vi "Untitled 1.vi"() -> ()   [LabVIEW 2025]
uses:
  <vilib>/Utility/error.llb/DialogType.ctl
  channel parameters cluster.ctl
  <resource>/objmgr/daqmx.rc
  <vilib>/DAQmx/write.llb/DAQmx Write (Analog 1D Wfm NChan NSamp).vi
  <vilib>/DAQmx/write.llb/DAQmx Write (Analog 1D DBL NChan 1Samp).vi
panel:
  in  "Galvo voltage":dbl
  in  "Galvo frequency":u16
  in  "Pulse Duty Cycle":dbl
  in  "Zelux Frequency":u16
  in  "488 nm LED control":dbl(slide) step=1.0 scale=0.0..100.0 scale format="%#_3g"
  in  "594 nm laser control":dbl(slide) step=1.0 scale=0.0..100.0 scale format="%#_3g"
  in  "Run Live":bool caption="Run live"
  out "594 changed":bool=TRUE
  out "488 changed":bool=TRUE
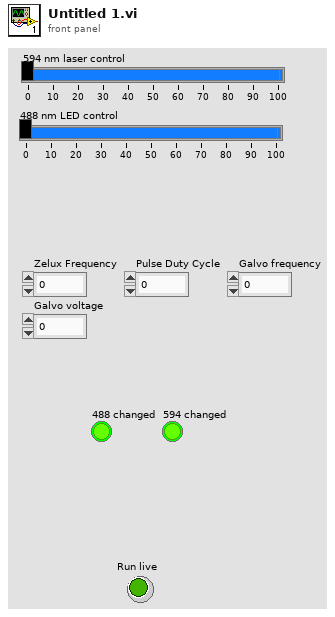
[diagram p1: front panel]
types:
  T1 = typedef "DialogType.ctl" = u16
  T2 = typedef "channel parameters cluster.ctl" = cluster{"voltage":dbl, "frequency":dbl, "duty cycle":dbl, "sample rate":dbl}
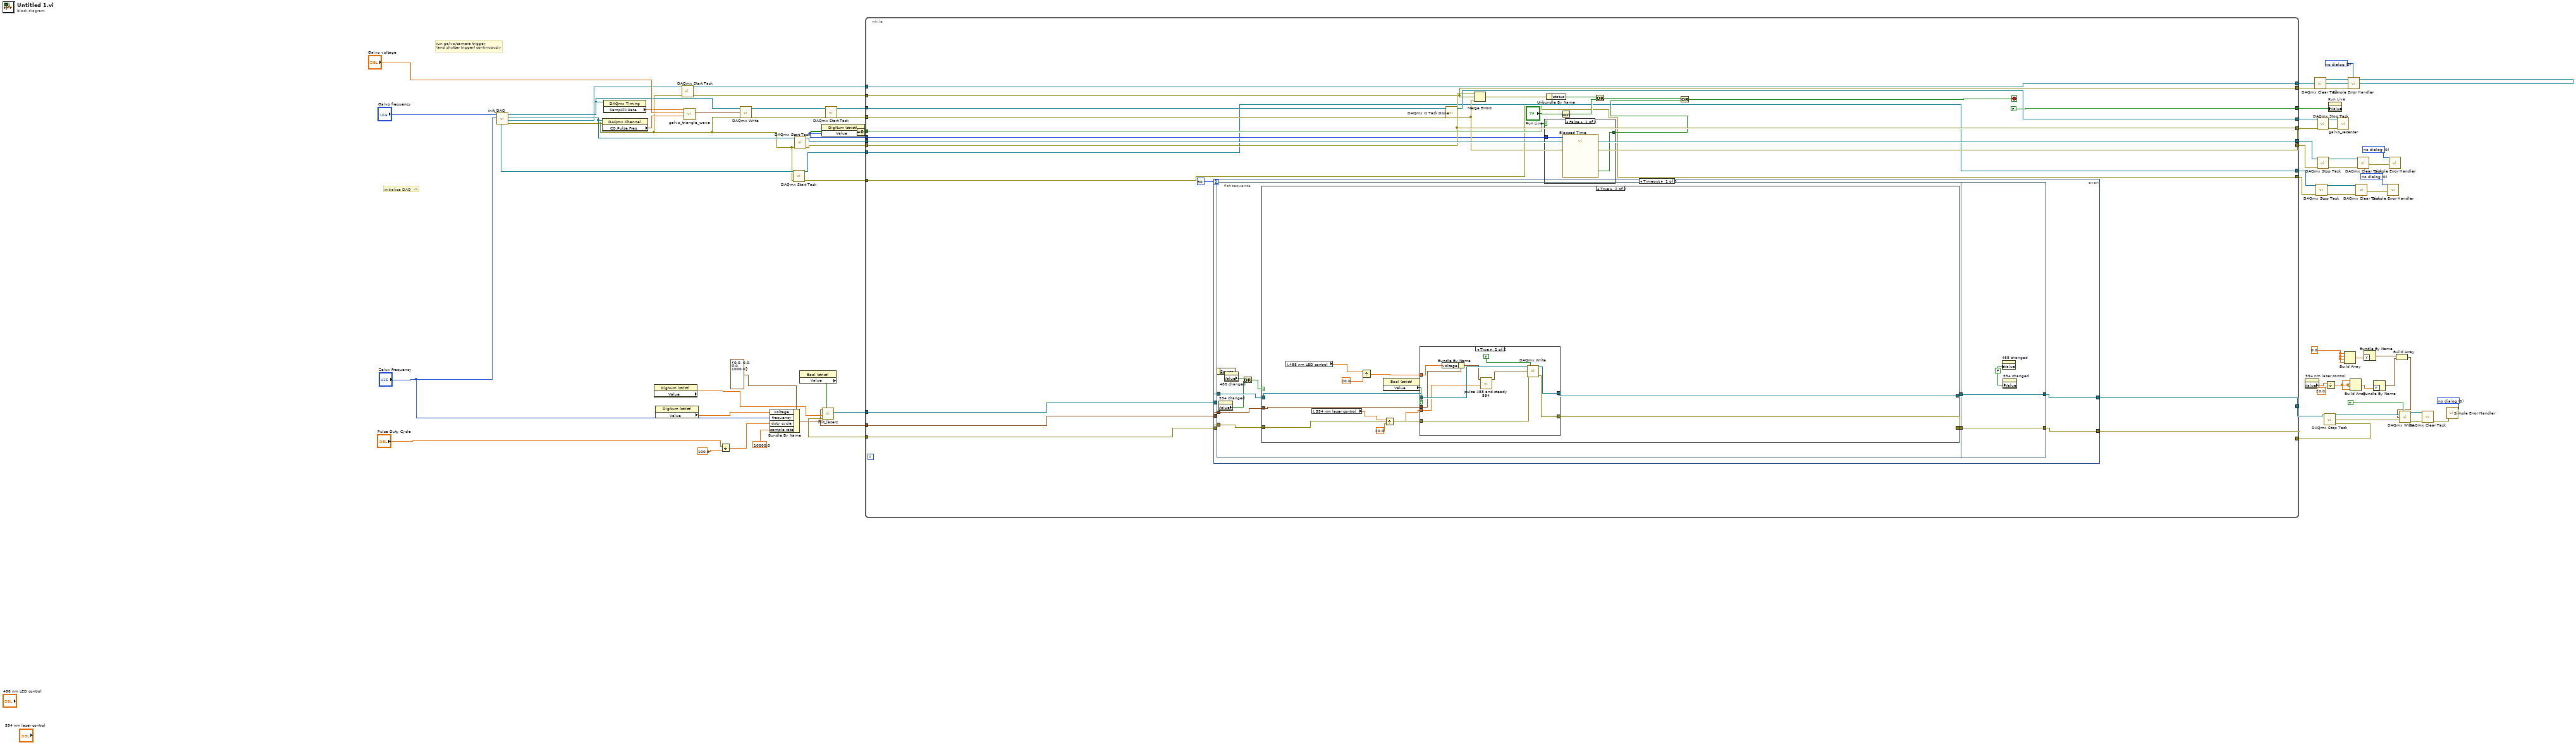
[diagram p0: block diagram]
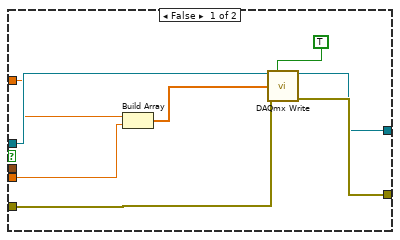
[diagram p3: hidden frame]
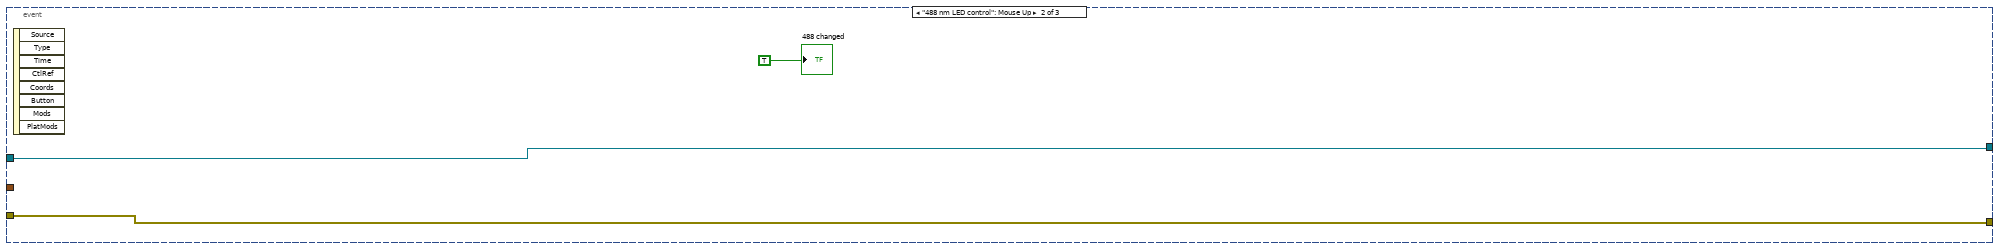
[diagram p4: hidden frame]
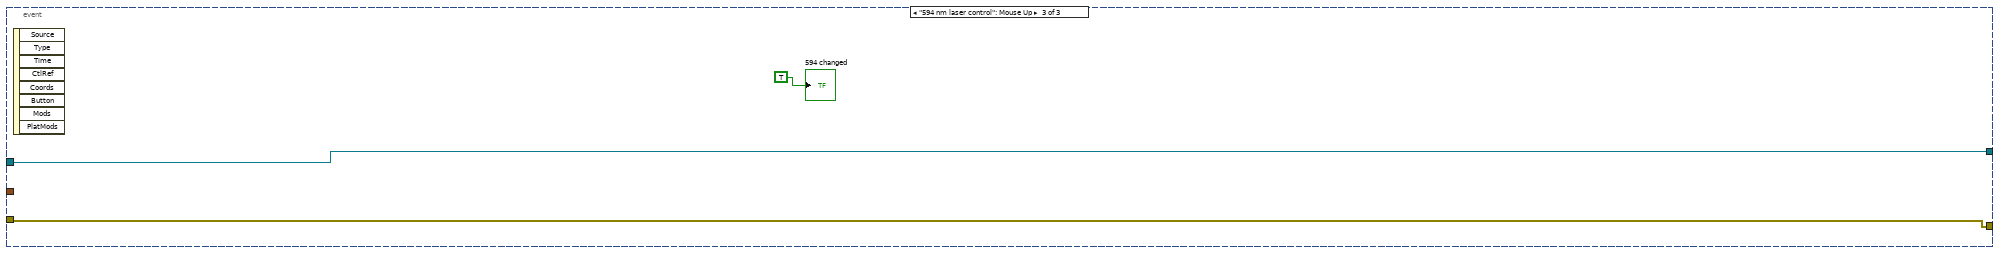
[diagram p5: hidden frame]
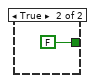
[diagram p6: hidden frame]
diagram:
  w5 = T1 0 items=["no dialog", "OK message", "continue or stop message", "OK message + warnings", "continue/stop + warnings"] ("type of dialog (OK msg:1)")
  w16 = 0.0
  w32 = T1 0 items=["no dialog", "OK message", "continue or stop message", "OK message + warnings", "continue/stop + warnings"] ("type of dialog (OK msg:1)")
  w57 = T1 0 items=["no dialog", "OK message", "continue or stop message", "OK message + warnings", "continue/stop + warnings"] ("type of dialog (OK msg:1)")
  w59 = T1 0 items=["no dialog", "OK message", "continue or stop message", "OK message + warnings", "continue/stop + warnings"] ("type of dialog (OK msg:1)")
  # "initialize DAQ  ->"
  # "run galvo/camera trigger \n(and shutter trigger) continuously"
  n1 = call "init_DAQ.vi"("Slow/Zelux frame frequency"="Zelux Frequency", "Fast/Kinetix frame frequency"="Galvo frequency") -> ("error out"=w9:errorcluster, "shutter trigger task"=w52:refnum<k21>, "Kinetix trigger task"=w47:refnum<k21>, "galvo driving task"=w63:refnum<k21>, "Zelux trigger task"=w10:refnum<k21>)  [unwired: 3 in, 2 out]
  n2 = property class="DAQmx Channel"(reference=w47, error in=w9) -> ("CO.Pulse.Freq"=w40:dbl)  [unwired: 2 out]
  n3 = property class="DAQmx Timing"(reference=w63) -> ("SampClk.Rate"=w39:dbl)  [unwired: 1 in, 2 out]
  n4 = property on="Property Node" class="DigNum (strict)"() -> ("Value"=w21:dbl)  [unwired: 2 in, 2 out]
  n5 = property on="Property Node" class="DigNum (strict)"() -> ("Value"=w22:dbl)  [unwired: 2 in, 2 out]
  n6 = call <vilib>:"DAQmx Start Task.vi"("task/channels in"=w52, "error in"=w9) -> ("task out"=w56:refnum<k21>, "error out"=w54:errorcluster)  [unwired: 12 in]
  n7 = call "galvo_triangle_wave.vi"("final frequency"=w40, "amplitude"="Galvo voltage", "sample rate"=w39) -> ("waveform array out"=w46:waveform(dbl)[])  [unwired: 8 in]
  n8 = Divide(x="Pulse Duty Cycle", y=100.0) -> (x/y=w25:dbl)
  n9 = call-poly <vilib>:"DAQmx Write.vi"("task/channels in"=w63, "data"=w46, "error in"=w9) -> ("task out"=w69:refnum<k21>, "error out"=w68:errorcluster)  [unwired: 10 in, 1 out]
  n10 = Bundle By Name(cluster=T2 {"voltage"=0.0, "frequency"=0.0, "duty cycle"=0.0, "sample rate"=1000.0} ("channel parameters"), "voltage"=w22, "frequency"="Zelux Frequency", "duty cycle"=w25, "sample rate"=10000.0) -> (w20:T2)
  n11 = call <vilib>:"DAQmx Start Task.vi"("task/channels in"=w10, "error in"=w9) -> ("task out"=w8:refnum<k21>, "error out"=w7:errorcluster)  [unwired: 12 in]
  n12 = call <vilib>:"DAQmx Start Task.vi"("task/channels in"=w47, "error in"=w9) -> ("task out"=w62:refnum<k21>, "error out"=w61:errorcluster)  [unwired: 12 in]
  n13 = property on="Property Node" class="Bool (strict)"() -> ("Value"=w27:bool)  [unwired: 2 in, 2 out]
  n14 = property on="Property Node" class="DigNum (strict)"() -> ("Value"=w42:i32)  [unwired: 2 in, 2 out]
  n15 = call "init_lasers.vi"("488 pulsed"=w27, "594 nm voltage"=w21, "488 nm channel parameters"=w20) -> ("error out"=w37:errorcluster, "task out"=w38:refnum<k21>)  [unwired: 6 in, 1 out]
  n16 = call <vilib>:"DAQmx Start Task.vi"("task/channels in"=w69, "error in"=w68) -> ("task out"=w64:refnum<k21>, "error out"=w65:errorcluster)  [unwired: 12 in]
  n17 = Equal To 0?(x=w42) -> (x = 0?=w43:bool)
  n18 = while {
    tunnel: w64 -> [w99]
    tunnel: w65 -> [w98]
    tunnel: [w88] -> w67
    tunnel: [w97] -> w66
    tunnel: w62 -> [w95]
    tunnel: w61 -> [w90]
    tunnel: [w90] -> w51
    tunnel: [w95] -> w49
    tunnel: w56 -> [w92]
    tunnel: [w92] -> w55
    tunnel: w54 -> [w89]
    tunnel: [w89] -> w53
    tunnel: w43 -> [w84]
    tunnel: w42 -> [w83]
    tunnel: [FALSE] -> w41
    tunnel: w38 -> [w81]
    tunnel: w37 -> [w80]
    tunnel: [w79] -> w36
    tunnel: [w78] -> w35
    tunnel: w20 -> [w76]
    tunnel: [w75] -> w2
    tunnel: w8 -> [w75]
    tunnel: [w74] -> w1
    tunnel: w7 -> [w74]
    stop <- w82 stop-if-true
    n19 = event shown="[0] Timeout" {
      selector: _ -> [_ _ _]
      dyn-events: _ -> [_ _ _]
      timeout: 50 -> [_ _ _]
      tunnel: w80 -> [w106 w151 w154]
      tunnel: [w100 w150 w153] -> w79
      tunnel: [w105 w151 w154] -> w78
      tunnel: w81 -> [w104 w150 w153]
      tunnel: w76 -> [w103 _ _]
      event Timeout {
        n20 = flat-sequence {
          tunnel: w106 -> [w114]
          tunnel: w104 -> [w112]
          tunnel: w103 -> [w107]
          tunnel: [w113] -> w102
          tunnel: [w108] -> w101
          tunnel: [w148] -> w100
          tunnel: [w149] -> w105
          tunnel: w102 -> [w149]
          tunnel: w101 -> [w148]
          frame #0 {
            n21 = property on="594 changed" class="Bool (strict)"() -> ("Value"=w109:bool)  [unwired: 2 in, 2 out]
            n22 = property on="488 changed" class="Bool (strict)"() -> ("Value"=w110:bool)  [unwired: 2 in, 2 out]
            n23 = Or(x=w110, y=w109) -> (x .or. y?=w111:bool)
            n24 = case shown="True" w111 {
              tunnel: w114 -> [w116 w127]
              tunnel: [w115 w126] -> w108
              tunnel: [w116 w125] -> w113
              tunnel: w112 -> [w115 w122]
              tunnel: w107 -> [_ w119]
              frame False {
              }
              frame True {
                n25 = local read "488 nm LED control"() -> (w118:dbl)
                n26 = local read "594 nm laser control"() -> (w117:dbl)
                n27 = Divide(x=w118, y=20.0) -> (x/y=w124:dbl)
                n28 = property on="Property Node" class="Bool (strict)"() -> ("Value"=w128:bool)  [unwired: 2 in, 2 out]
                n29 = Divide(x=w117, y=20.0) -> (x/y=w123:dbl)
                n30 = case shown="True" w128 {
                  tunnel: [w136 w143] -> w125
                  tunnel: w127 -> [w135 w144]
                  tunnel: w122 -> [w133 w145]
                  tunnel: [w134 w146] -> w126
                  tunnel: w124 -> [w131 w139]
                  tunnel: w123 -> [w130 w141]
                  tunnel: w119 -> [_ w138]
                  frame False {
                    n31 = Build Array(w131, w130) -> (w129:dbl[])
                    n32 = call-poly <vilib>:"DAQmx Write.vi"("task/channels in"=w133, "auto start"=TRUE, "data"=w129, "error in"=w135) -> ("task out"=w134:refnum<k21>, "error out"=w136:errorcluster)  [unwired: 9 in, 1 out]
                  }
                  frame True {
                    n33 = Bundle By Name(cluster=w138, "voltage"=w139) -> (w137:T2)
                    n34 = call "pulse 488 and steady 594.vi"("594 amplitude"=w141, "488 nm channel parameters"=w137) -> ("waveforms out"=w140:waveform(dbl)[])  [unwired: 9 in]
                    n35 = call-poly <vilib>:"DAQmx Write.vi"("task/channels in"=w145, "auto start"=TRUE, "data"=w140, "error in"=w144) -> ("task out"=w146:refnum<k21>, "error out"=w143:errorcluster)  [unwired: 9 in, 1 out]
                  }
                }
              }
            }
          }
          frame #1 {
            w147 = FALSE ("488 changed")
            n36 = property on="488 changed" class="Bool (strict)"("Value"=w147) -> ()  [unwired: 2 in, 2 out]
            n37 = property on="594 changed" class="Bool (strict)"("Value"=w147) -> ()  [unwired: 2 in, 2 out]
          }
        }
        n38 = event-data() -> ()  [unwired: 1 in, 1 out]
      }
      event "488 nm LED control": Mouse Up {
        n39 = event-data() -> ()  [unwired: 1 in, 8 out]
        "488 changed" <- TRUE ("488 changed")
      }
      event "594 nm laser control": Mouse Up {
        n40 = event-data() -> ()  [unwired: 1 in, 8 out]
        "594 changed" <- TRUE
      }
    }
    n41 = call <vilib>:"DAQmx Is Task Done.vi"("task/channels in"=w99, "error in"=w98) -> ("task out"=w97:refnum<k21>, "error out"=w88:errorcluster)  [unwired: 11 in, 1 out]
    n42 = Merge Errors(w90, w89, w88) -> (w91:errorcluster)
    n43 = case shown="False" w84 {
      tunnel: [w157 FALSE] -> w86
      tunnel: w83 -> [w156 _]
      frame False {
        n44 = call "Elapsed Time"("Time Target (s)"=w156) -> ("Time has Elapsed"=w157:bool)  [unwired: 11 in, 7 out]
      }
      frame True {
      }
    }
    n45 = Unbundle By Name(w91) -> ("status"=w96:bool)
    n46 = Not(x="Run Live") -> (.not. x?=w94:bool)
    n47 = Or(x=w96, y=w94) -> (x .or. y?=w87:bool)
    n48 = Or(x=w87, y=w86) -> (x .or. y?=w82:bool)
  }
  n49 = property on="594 nm laser control" class="Slide (strict)"() -> ("Value"=w15:dbl)  [unwired: 2 in, 2 out]
  n50 = call <vilib>:"DAQmx Clear Task.vi"("task in"=w55, "error in"=w53) -> ("error out"=w58:errorcluster)  [unwired: 13 in]
  n51 = call <vilib>:"DAQmx Stop Task.vi"("task/channels in"=w2, "error in"=w1) -> ("task out"=w3:refnum<k21>, "error out"=w4:errorcluster)  [unwired: 12 in]
  n52 = call <vilib>:"DAQmx Stop Task.vi"("task/channels in"=w66, "error in"=w67) -> ("task out"=w45:refnum<k21>, "error out"=w44:errorcluster)  [unwired: 12 in]
  n53 = call <vilib>:"DAQmx Stop Task.vi"("task/channels in"=w49, "error in"=w51) -> ("task out"=w48:refnum<k21>, "error out"=w50:errorcluster)  [unwired: 12 in]
  n54 = call <vilib>:"DAQmx Stop Task.vi"("task/channels in"=w36, "error in"=w35) -> ("task out"=w33:refnum<k21>, "error out"=w34:errorcluster)  [unwired: 12 in]
  n55 = Divide(x=w15, y=20.0) -> (x/y=w13:dbl)
  n56 = property on="Run Live" class="Bool (strict)"("Value"=w41) -> ()  [unwired: 2 in, 2 out]
  n57 = call "galvo_recenter.vi"("error in"=w44, "task/channels in"=w45) -> ()  [unwired: 10 in]
  n58 = Build Array(w16, w16, w16, w16) -> (w18:dbl[])
  n59 = call <vilib>:"Simple Error Handler.vi"("type of dialog (OK msg:1)"=w57, "error in (no error)"=w58) -> ()  [unwired: 3 in, 5 out]
  n60 = Build Array(w13, w13, w13, w13) -> (w12:dbl[])
  n61 = call <vilib>:"DAQmx Clear Task.vi"("task in"=w3, "error in"=w4) -> ("error out"=w6:errorcluster)  [unwired: 13 in]
  n62 = call <vilib>:"DAQmx Clear Task.vi"("task in"=w48, "error in"=w50) -> ("error out"=w60:errorcluster)  [unwired: 13 in]
  n63 = Bundle By Name("Y"=w18) -> (w19:waveform(dbl))  [unwired: 1 in]
  n64 = Bundle By Name("Y"=w12) -> (w11:waveform(dbl))  [unwired: 1 in]
  n65 = call <vilib>:"Simple Error Handler.vi"("type of dialog (OK msg:1)"=w5, "error in (no error)"=w6) -> ()  [unwired: 3 in, 5 out]
  n66 = call <vilib>:"Simple Error Handler.vi"("type of dialog (OK msg:1)"=w59, "error in (no error)"=w60) -> ()  [unwired: 3 in, 5 out]
  n67 = Build Array(w19, w11) -> (w17:waveform(dbl)[])
  n68 = call-poly <vilib>:"DAQmx Write.vi"("task/channels in"=w33, "auto start"=TRUE, "data"=w17, "error in"=w34) -> ("task out"=w30:refnum<k21>, "error out"=w29:errorcluster)  [unwired: 9 in, 1 out]
  n69 = call <vilib>:"DAQmx Clear Task.vi"("task in"=w30, "error in"=w29) -> ("error out"=w31:errorcluster)  [unwired: 13 in]
  n70 = call <vilib>:"Simple Error Handler.vi"("type of dialog (OK msg:1)"=w32, "error in (no error)"=w31) -> ()  [unwired: 3 in, 5 out]
